vi "Register for Waveform Data Events (CDB).vi"(8 "error in (no error)":errorcluster, 10 "WaveformStreamSpecifications":T3[](array[typedef]), 11 "WaveformStreaming in":T4) -> (0 "error out":errorcluster, 3 "WaveformStreaming out":T4, 4 "waveform data event registration (CDB)":refnum<event-registration>, 5 "registered waveform data event (CDB)":T1)   [LabVIEW 2020, in "NI_VS Waveform Streaming Interface.lvlib"]
doc: "Registers to receive waveform data from the specified <B>WaveformStreamSpecifications</B>. You can use this VI prior to starting waveform streams to generate an event registration refnum that allows an Event structure to stream data from waveforms. You must manually select the instance to use."
uses:
  <vilib>/NI VeriStand/Execution/WaveformStreaming/NI_VS Waveform Streaming Interface.lvlib
  <vilib>/NI VeriStand/Execution/WaveformStreaming/WaveformStreamingAPI.ctl
  NationalInstruments.VeriStand.ClientAPI
  <vilib>/NI VeriStand/Execution/WaveformStreaming/WaveformStreamSpecification.ctl
  <vilib>/NI VeriStand/Execution/WaveformStreaming/Registered Waveform Streams Data Event Refnum (CDB).ctl
  <vilib>/NI VeriStand/Execution/WaveformStreaming/Waveform Data Watcher Event Data (CDB).ctl
  <vilib>/NI VeriStand/Execution/WaveformStreaming/WaveformDataWatcherCDB.ctl
  <vilib>/NI VeriStand/Execution/WaveformStreaming/WaveformDataEventHandler Event Callback (CDB).vi
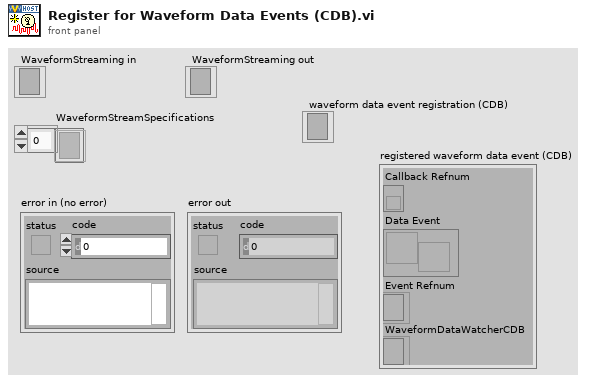
[diagram p1: front panel]
types:
  T1 = typedef "NI_VS Waveform Streaming Interface.lvlib/Registered Waveform Streams Data Event Refnum (CDB).ctl" = cluster{"Callback Refnum":refnum<k27>, "Data Event":refnum<user-event>, "Event Refnum":refnum<event-registration>, "WaveformDataWatcherCDB":T2}
  T2 = typedef "NI_VS Waveform Streaming Interface.lvlib/WaveformDataWatcherCDB.ctl" = refnum<k24>
  T3 = typedef "NI_VS Waveform Streaming Interface.lvlib/WaveformStreamSpecification.ctl" = refnum<k24>
  T4 = typedef "NI_VS Waveform Streaming Interface.lvlib/WaveformStreamingAPI.ctl" = refnum<k24>
  T5 = typedef "NI_VS Waveform Streaming Interface.lvlib/Waveform Data Watcher Event Data (CDB).ctl" = cluster{"Data":cdb[], "dt":dbl, "offset from start (samples)":u64, "t0 at start":timestamp, "WaveformStreamSpecification":T3}
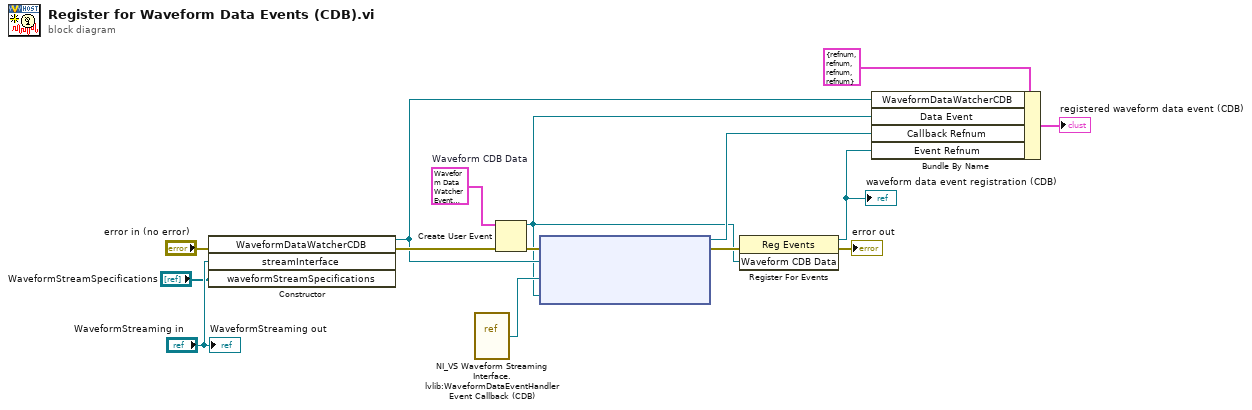
[diagram p0: block diagram]
diagram:
  w4 = T5 {"Data"=[], "dt"=0.0, "offset from start (samples)"=0, "t0 at start"=timestamp(0 s since 1904-01-01), "WaveformStreamSpecification"=refnum}  # Waveform CDB Data
  n1 = constructor class="WaveformDataWatcherCDB"(error in="error in (no error)", "streamInterface"="WaveformStreaming in", "waveformStreamSpecifications"="WaveformStreamSpecifications") -> (reference out=w5:refnum<k24>, error out=w13:errorcluster)  [unwired: 2 in, 3 out]
  n2 = vi-ref "NI_VS Waveform Streaming Interface.lvlib:WaveformDataEventHandler Event Callback (CDB).vi"() -> (w6:refnum<vi>)
  n3 = Create User Event(user event datatype=w4, error in=w13) -> (user event=w3:refnum<user-event>, error out=w12:errorcluster)
  n4 = node(w12, w5, w6, w3) -> (w7:refnum<k27>, w11:errorcluster)  [unwired: 1 in]
  n5 = register-events(error in=w11, w3) -> (reference out=w2:refnum<event-registration>, error out=→"error out":errorcluster)  [unwired: 1 in]
  "waveform data event registration (CDB)" <- w2
  n6 = Bundle By Name(cluster=T1 {"Callback Refnum"=refnum, "Data Event"=refnum, "Event Refnum"=refnum, "WaveformDataWatcherCDB"=refnum} ("Registered DBL Waveform Streams Data Event Refnum"), "WaveformDataWatcherCDB"=w5, "Data Event"=w3, "Callback Refnum"=w7, "Event Refnum"=w2) -> (→"registered waveform data event (CDB)":T1)
  "WaveformStreaming out" <- "WaveformStreaming in"
